vi "Dashboard Main.vi"() -> ()   [LabVIEW 2014]
uses:
  Program Files (x86)/National Instruments/LabVIEW 2014/examples/FRC/roboRIO/Vision/2015 Vision Example/Vision Support Code/Camera Types.ctl
  <vilib>/event_ctls.llb/eventvkey.ctl
  <vilib>/Rock Robotics/WPI/Dashboard/WPI_DashboardLogging Global.vi
  <vilib>/Rock Robotics/Network Tables/SD Write Number.vi
  <vilib>/Utility/config.llb/Write Key (String).vi
  <vilib>/Utility/config.llb/Write Key (I32).vi
  <vilib>/Utility/config.llb/NI_LVConfig.lvlib
  <vilib>/vision/NI_Vision_Development_Module.lvlib
panel:
  out "Camera Image 6":T1(plugin-control)
  in  "Tab Control":enum32{"Original", "Masked"}(tab)
  out "Original Image":T1(plugin-control)
  out "Masked":T1(plugin-control)
  out "Image Message":string="Timeout in Camera Communications"
  in  "TCP":refnum<k5>
  in  "Rec Mode":enum32{"Stop", "Record", "Playback"}(radio)
  in  "Vision":u16(ring)=3 items=["Camera Off", "USB Camera SW", "USB Camera HW", "IP Camera"]
  out "Camera IP":string
  in  "Dashboard Tab":T2(tab)
  in  "Camera Settings":T3={"Frame Rate"=30, "Compression"=30, "Size"=1} {"Frame Rate" scale=1.0..30.0; "Size" items=["640x480", "320x240", "160x120"]}
  out "MotorChart R":cluster{"Numeric":dbl, "Numeric":dbl}(graph)
  out "MotorChart L":T4(graph)
  out "MotorSliders R":cluster{"MotorSlide1":dbl, "MotorSlide2":dbl} {"MotorSlide2" scale=-1.0..1.0 scale format="%#_2e"; "MotorSlide1" scale=-1.0..1.0 scale format="%#_2e"}
  out "MotorSliders L":T5 {"MotorSlide4 2" scale=0.0..14.0 scale format="%#_2e"; "MotorSlide2" scale=-1.0..1.0 scale format="%#_2e"; "MotorSlide1" scale=-1.0..1.0 scale format="%#_2e"}
  out "Gyro":dbl(knob) scale=0.0..360.0
  out "JS1 Z":dbl(slide) scale=-1.0..1.0 scale format="%#_2e"
  out "JS1 Graph":cluster{"X":dbl, "Y":dbl}[](graph)
  out "JS1 Buttons":T6
  out "JS2 Z":dbl(slide) scale=-1.0..1.0 scale format="%#_2e"
  out "JS2 Graph":cluster{"X":dbl, "Y":dbl}[](graph)
  out "JS2 Buttons":T6
  out "Mode":T7(ring)=enum."Auto Disabled"
  in  "DB Camera Config":bool
  out "fps":dbl format="%#.1g"
  out "Mbps":dbl format="%#.1g"
  out "Mbps 2":bool
  out "Center":dbl
  out "Sorted Scores":T8(array[cluster]) {"Carpet" format="%#_3g"; "S" format="%#_3g"; "Trapezoid %" format="%#_3g"; "L" format="%#_3g"; "Area to CH" format="%#_3g"; "X" format="%#_3g"; "Y" format="%#_3g"}
  out "Detected Totes":T9(array[cluster]) {"Normalized Rect"."Numeric 5" format="%#_2g"; "Normalized Rect"."Numeric 3" format="%#_2g"; "Normalized Rect"."Numeric 2" format="%#_2g"; "Normalized Rect"."Numeric" format="%#_2g"}
  out "ms to process":u32
  in  "Tote Color":T10={"Hue"={23.67058792990901, 53.0}, "Sat"={88.0, 255.0}, "Val"={60.0, 159.85714285714286}} {"Hue" scale=0.0..255.0 scale format="%#_3g"}
  in  "Carpet Color":T11(tab)
  in  "Red":T10={"Hue"={231.0, 14.0}, "Sat"={83.0, 255.0}, "Val"={52.5, 255.0}} {"Hue" scale=0.0..255.0 scale format="%#_3g"}
  in  "Blue":T10={"Hue"={119.0, 181.0}, "Sat"={33.0, 255.0}, "Val"={48.571428571428584, 255.0}} {"Hue" scale=0.0..255.0 scale format="%#_3g"}
  in  "Annotate":bool=TRUE
  in  "Show Carpet Mask":bool=TRUE
  in  "Limit Tests?":bool=TRUE
  out "Particles":i32
  in  "Score Threshold":dbl=75.0
  in  "Aspect Fudge Factor":dbl=1.0
  in  "Camera Type":T12=enum."MS HD3000 square"
  out "Image":T1(plugin-control)
  in  "DB/String 9":string
  in  "DB/String 8":string
  in  "DB/String 7":string
  in  "DB/String 6":string
  in  "DB/String 5":string
  in  "DB/String 4":string
  in  "DB/String 3":string
  in  "DB/String 2":string
  in  "DB/String 1":string
  in  "DB/String 0":string
  in  "DB/Slider 0":dbl(slide) scale=0.0..5.0
  in  "DB/Slider 1":dbl(slide) scale=0.0..5.0
  in  "DB/Slider 2":dbl(slide) scale=0.0..5.0
  in  "DB/Slider 3":dbl(slide) scale=0.0..5.0
  out "DB/LED 3":bool
  out "DB/LED 2":bool
  out "DB/LED 1":bool
  out "DB/LED 0":bool
  in  "DB/Button 3":bool
  in  "DB/Button 2":bool
  in  "DB/Button 1":bool
  in  "DB/Button 0":bool caption="New Name"
  in  "Test Slider":dbl(slide) scale=0.0..100.0 scale format="%#_3g"
  in  "On/Off":bool caption="Solenoid"
  in  "Test Name":u16(ring) items=["Select the test to run...", "Example Test", "-------------------------------", "List of tests is built in robot code.", "Replace with your own automated tests."]
  in  "Test Tree":string(tree)
  in  "Motor":cluster{"Value":dbl, "Enable":bool} {"Value" scale=-1.0..1.0 scale format="%#_3g"}
  out "Progress":T13 {"Test Progress" scale=0.0..100.0}
  in  "Rev/Fwd":cluster{"Forward":bool, "Reverse":bool}
  in  "Test Ring":u16(ring) items=["Monochrome", "Color"]
  in  "Listbox":i32(listbox)
  out "Tree":string(tree)
  out "Boolean":bool
  # "Left"
  # "Front"
  # "Right"
  # "Battery"
  # "Density Profile"
  # "Aspect Ratio"
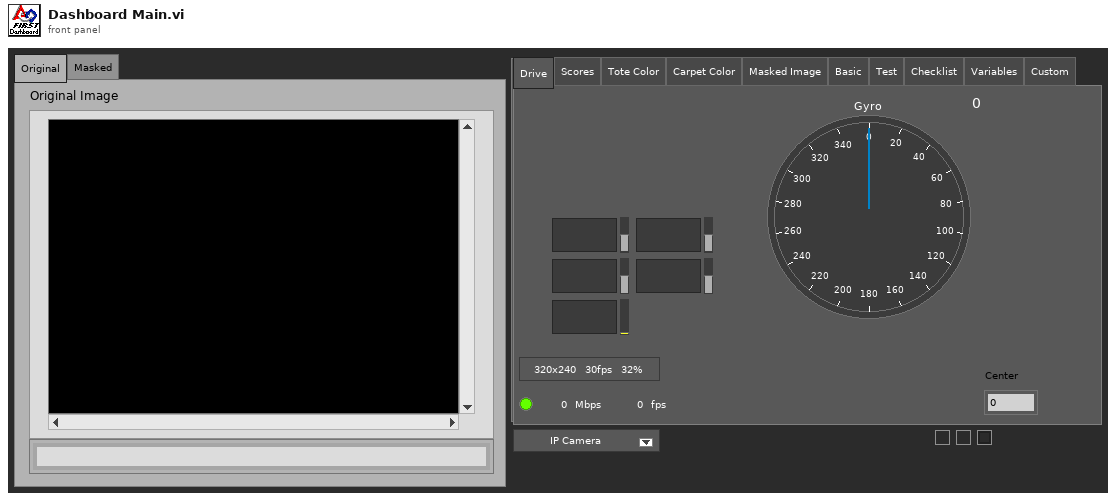
[diagram p1: front panel]
types:
  T1 = typedef "IMAQ Image.ctl" = refnum<image>
  T2 = enum32{"Drive", "Scores", "Tote Color", "Carpet Color", "Masked Image", "Basic", "Test", "Checklist", "Variables", "Custom"}
  T3 = cluster{"Frame Rate":i32, "Compression":i32, "Size":u16}
  T4 = cluster{"Numeric":dbl, "Numeric":dbl, "Battery V":dbl}
  T5 = cluster{"MotorSlide1":dbl, "MotorSlide2":dbl, "MotorSlide4 2":dbl}
  T6 = cluster{bool, bool, bool, bool, bool, bool, bool, bool, bool, bool, bool, bool}
  T7 = enum8{"Tele-Op Disabled", "Tele-Op Enabled", "Auto Disabled", "Auto Enabled", "Test Disabled", "Test Enabled", "Disconnected", "No Code", "E-Stop"}
  T8 = cluster{"Rectangle":cluster{"Numeric":dbl, "Numeric 2":dbl, "Numeric 3":dbl, "Numeric 5":dbl}, "Trapezoid %":dbl, "L":dbl, "S":dbl, "Area to CH":dbl, "X":dbl, "Y":dbl, "Carpet":dbl}[]
  T9 = cluster{"Distance (ft)":dbl, "Center":cluster{dbl, dbl}, "Normalized Rect":cluster{"Numeric":dbl, "Numeric 2":dbl, "Numeric 3":dbl, "Numeric 5":dbl}}[]
  T10 = cluster{"Hue":cluster{dbl, dbl}, "Sat":cluster{dbl, dbl}, "Val":cluster{dbl, dbl}}
  T11 = enum32{"Red Carpet Color", "Blue Carpet Color", "None"}
  T12 = typedef "Camera Types.ctl" = enum16{"206", "1011", "1013", "MS HD3000 square", "MS HD3000 640x480"}
  T13 = cluster{"Test Progress":u8, "Test Progress Text":string}
  T14 = typedef "Particle Parameters" = i32
  T15 = typedef "Image Type" = u32
  T16 = enum32{"Drive", "Basic", "Custom", "Test", "Checklist", "Variables"}
  T17 = cluster{"Camera Image 6":refnum<vi>, "Dashboard Tab":refnum<vi>, "Boolean":refnum<vi>, "Vision":refnum<vi>, "Rec Mode":refnum<vi>, "Test Slider":refnum<vi>, "On/Off ":refnum<vi>, "Test Ring":refnum<vi>, "Rev/Fwd":refnum<vi>, "Test Name":refnum<vi>, "Motor":refnum<vi>, "Progress":refnum<vi>, "CheckList":refnum<vi>, "Tree":refnum<vi>, "Test Tree":refnum<vi>}
  T18 = cluster{"Error Strings":string, "Disable Counts":cluster{u16, u16}, "Rail Faults":cluster{u16, u16, u16}, "Robot IP":string, "DB Mode":u8, "Event Info":cluster{"Name":string, "Type":u8, "Number":u16, "Replay":u8}, "Camera Addr":string}
  T19 = cluster{"Storage":cluster{"Disk Free":u64, "RAM Block":u32, "RAM free":u32}, "CPU Utilization":cluster{"CPU % ISR":sgl, "CPU % Time Crit":sgl, "CPU % Timed Str":sgl, "CPU % High":sgl, "CPU % Above":sgl, "CPU % Normal":sgl, "CPU % Low":sgl}, "CAN":cluster{"% Bus Utilization":sgl, "Bus Off Cnt":u32, "TX_FIFO Full Cnt":u32, "Receive Error Cnt":u8, "Transmit Error Cnt":u8}, "HID":cluster{"HID Outputs":u32, "Rumble Low":u16, "Rumble High":u16}[]}
  T20 = cluster{"Status bits":cluster{"Test Mode":bool, "Autonomous":bool, "Enabled":bool, "Code Start":bool, "Brownout":bool, "Reserved 2":bool, "Reserved 3":bool, "E-Stop":bool}, "Code Trace":cluster{"Disabled":bool, "TeleOp":bool, "Auto":bool, "Test":bool}, "Controller Type":enum16{"unknown", "cRIO", "roboRio"}, "Code?":enum16{"unknown", "noCode", "code"}, "Battery V":dbl}
  T21 = cluster{"Control Bits":cluster{"TestMode":bool, "Autonomous":bool, "Enabled":bool, "FMS Present":bool, bool, bool, bool, "E-Stop":bool}, "Team Station ":u8, "Countdown":sgl, "Joystick Values":cluster{"Axes":dbl[], "Buttons":bool[], "POVs":i16[]}[]}
  T22 = cluster{"Axes":dbl[], "Buttons":bool[], "POVs":i16[]}[]
  T23 = cluster{"Axes":dbl[], "Buttons":bool[], "POVs":i16[]}
  T24 = cluster{"Buttons[0]":bool, "Buttons[1]":bool, "Buttons[2]":bool, "Buttons[3]":bool, "Buttons[4]":bool, "Buttons[5]":bool, "Buttons[6]":bool, "Buttons[7]":bool, "Buttons[8]":bool, "Buttons[9]":bool, "Buttons[10]":bool, "Buttons[11]":bool}
  T25 = typedef "NI_LVConfig.lvlib/Config Data RefNum.ctl" = refnum<k1>
  T26 = cluster{"Operation":enum16{"Update", "Clear"}, "Color Box":u32}[]
  T27 = typedef "eventvkey.ctl" = enum16{"ASCII", "Enter", "Return", "Shift", "Ctrl", "Alt", "Cmd", "Opt", "Caps", "NumLock", "Clear", "Break", "Up", "Down", "Left", "Right", "Insert", "Delete", "Home", "End", "PageUp", "PageDown", "Escape", "Help", "Pause", "ScrollLock", "F1", "F2", "F3", "F4", "F5", "F6", "F7", "F8", "F9", "F10", "F11", "F12", "F13", "F14", "F15", "F16", "F17", "F18", "F19", "F20", "F21", "F22", "F23", "F24", "Play", "VolumeUp", "VolumeDown", "Mute", "Two Byte Char"}
  T28 = cluster{"Image Size":bool, "Image Type":bool, "Pixel Value":bool, "ROI Information":bool, "Zoom Factor":bool}
  T29 = enum8{"Enabled", "Disabled", "Disabled and Grayed Out"}
  T30 = cluster{"Operation":enum16{"Update", "Clear"}, "Color Box":u32}
  T31 = cluster{"Bounding box":cluster{"left":dbl, "top":dbl, "right":dbl, "bottom":dbl}, "Trapezoid":dbl, "Long Aspect":dbl, "Short Aspect":dbl, "Area to CH":dbl, "X Mask":dbl, "Y Mask":dbl, "Carpet":dbl}[]
  T32 = cluster{"Red":cluster{"Hue":cluster{dbl, dbl}, "Sat":cluster{dbl, dbl}, "Val":cluster{dbl, dbl}}, "Blue":cluster{"Hue":cluster{dbl, dbl}, "Sat":cluster{dbl, dbl}, "Val":cluster{dbl, dbl}}}
  T33 = cluster{cluster{"[0]":dbl, "[1]":dbl, "[2]":dbl, "[3]":dbl}, "Score":dbl, "Long Edge Score":dbl, "Short Edge Score":dbl, dbl, "X Score":dbl, "Y Score":dbl, "Carpet":dbl}[]
  T34 = cluster{"Found Totes[0]":cluster{"Distance (ft)":dbl, "Center":cluster{dbl, dbl}, "Normalized Rect":cluster{"Numeric":dbl, "Numeric 2":dbl, "Numeric 3":dbl, "Numeric 5":dbl}}, "Found Totes[1]":cluster{"Distance (ft)":dbl, "Center":cluster{dbl, dbl}, "Normalized Rect":cluster{"Numeric":dbl, "Numeric 2":dbl, "Numeric 3":dbl, "Numeric 5":dbl}}, "Found Totes[2]":cluster{"Distance (ft)":dbl, "Center":cluster{dbl, dbl}, "Normalized Rect":cluster{"Numeric":dbl, "Numeric 2":dbl, "Numeric 3":dbl, "Numeric 5":dbl}}, "Found Totes[3]":cluster{"Distance (ft)":dbl, "Center":cluster{dbl, dbl}, "Normalized Rect":cluster{"Numeric":dbl, "Numeric 2":dbl, "Numeric 3":dbl, "Numeric 5":dbl}}, "Found Totes[4]":cluster{"Distance (ft)":dbl, "Center":cluster{dbl, dbl}, "Normalized Rect":cluster{"Numeric":dbl, "Numeric 2":dbl, "Numeric 3":dbl, "Numeric 5":dbl}}, "Found Totes[5]":cluster{"Distance (ft)":dbl, "Center":cluster{dbl, dbl}, "Normalized Rect":cluster{"Numeric":dbl, "Numeric 2":dbl, "Numeric 3":dbl, "Numeric 5":dbl}}, "Found Totes[6]":cluster{"Distance (ft)":dbl, "Center":cluster{dbl, dbl}, "Normalized Rect":cluster{"Numeric":dbl, "Numeric 2":dbl, "Numeric 3":dbl, "Numeric 5":dbl}}, "Found Totes[7]":cluster{"Distance (ft)":dbl, "Center":cluster{dbl, dbl}, "Normalized Rect":cluster{"Numeric":dbl, "Numeric 2":dbl, "Numeric 3":dbl, "Numeric 5":dbl}}, "Found Totes[8]":cluster{"Distance (ft)":dbl, "Center":cluster{dbl, dbl}, "Normalized Rect":cluster{"Numeric":dbl, "Numeric 2":dbl, "Numeric 3":dbl, "Numeric 5":dbl}}}
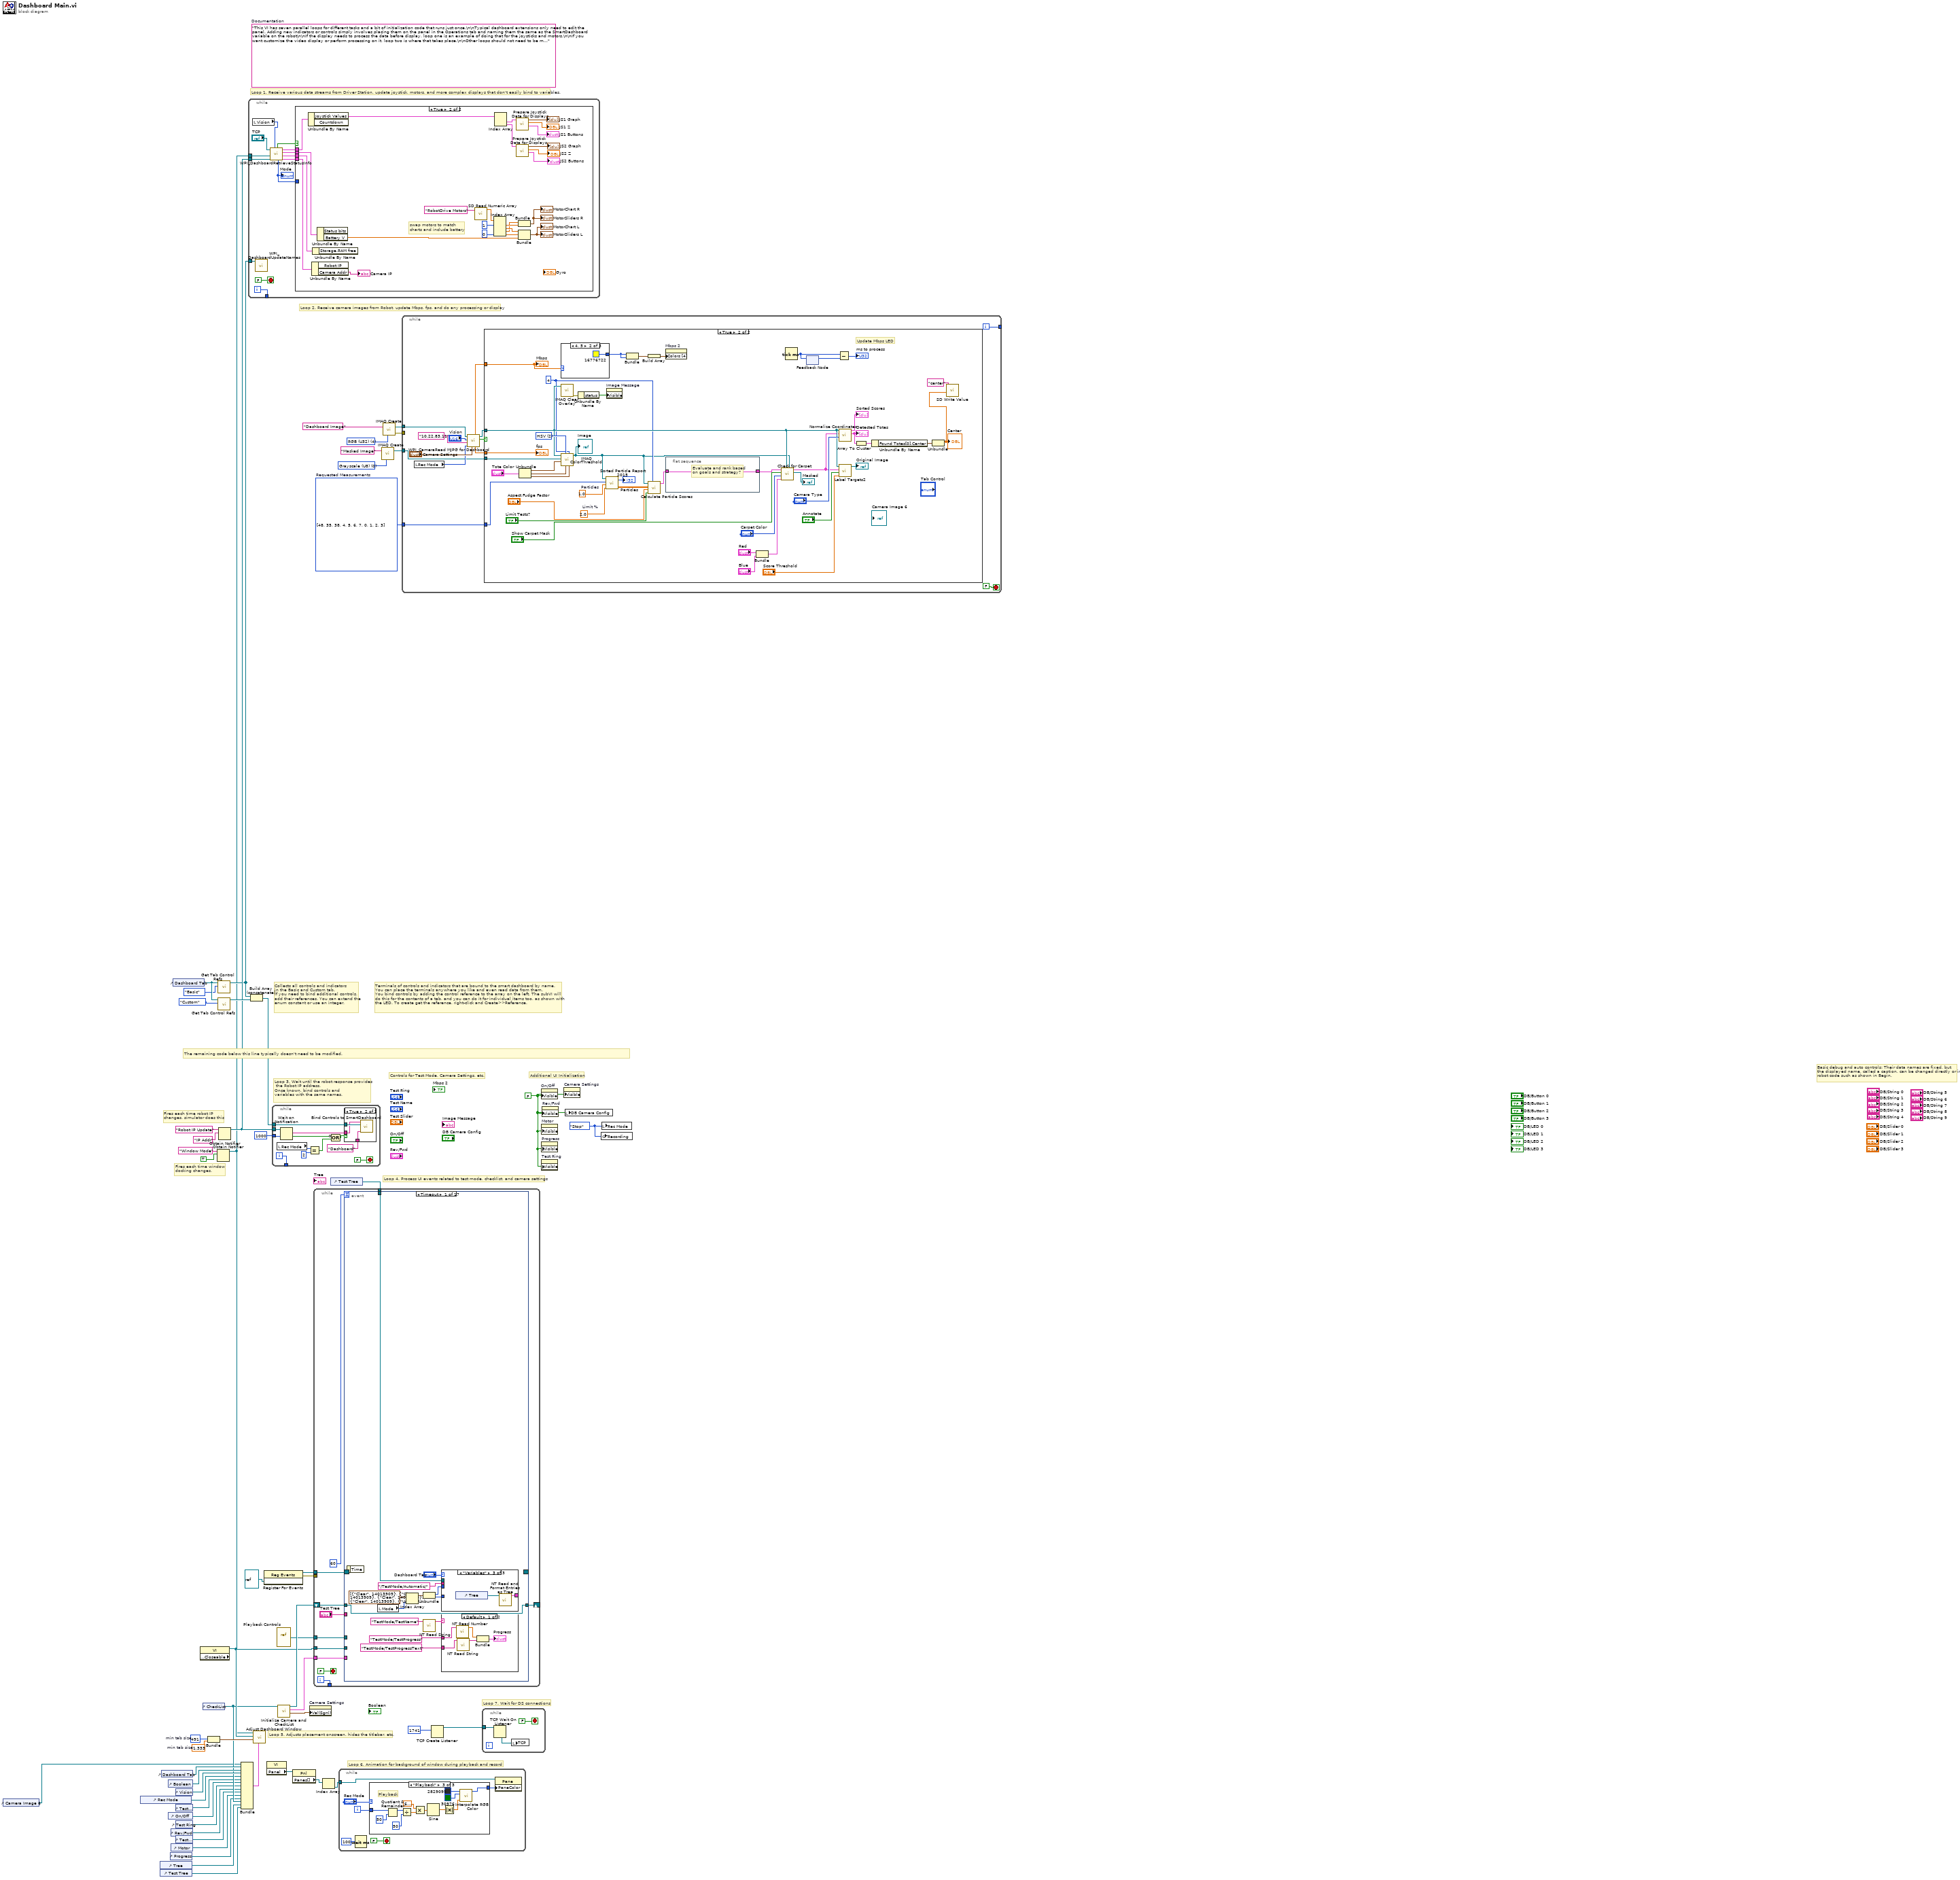
[diagram p0: block diagram]
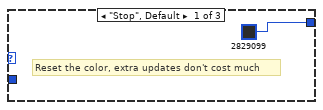
[diagram p3: hidden frame]
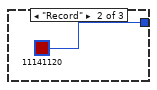
[diagram p4: hidden frame]
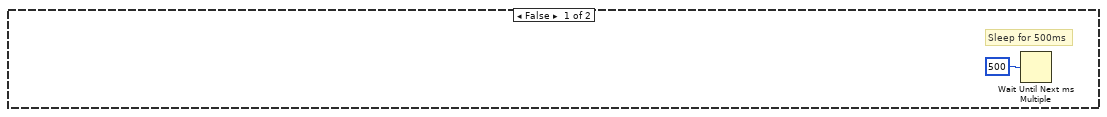
[diagram p6: hidden frame]
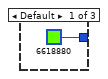
[diagram p7: hidden frame]
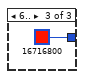
[diagram p8: hidden frame]
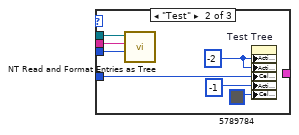
[diagram p10: hidden frame]
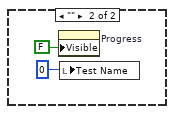
[diagram p11: hidden frame]
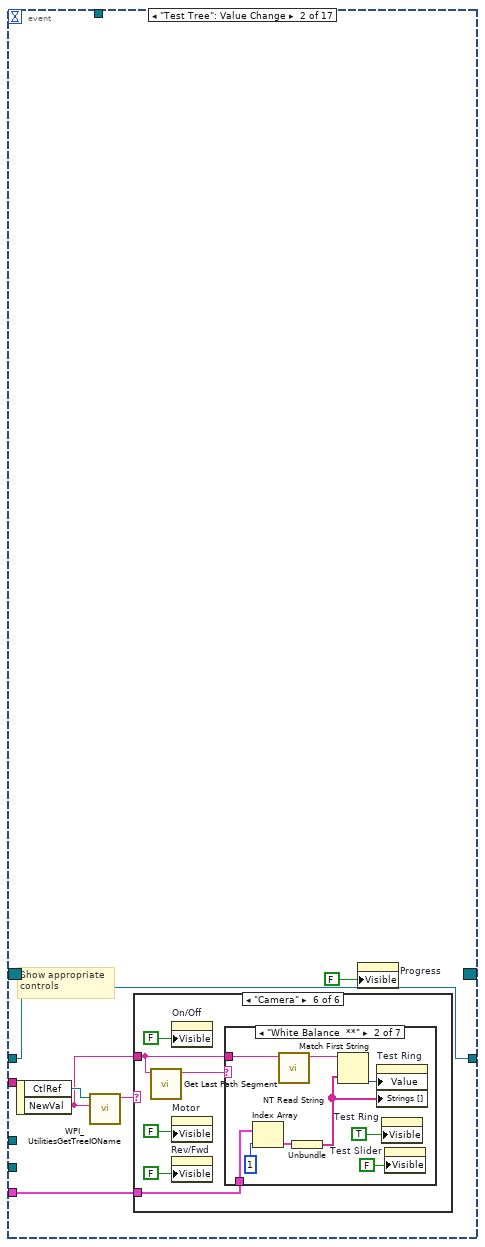
[diagram p12: hidden frame]
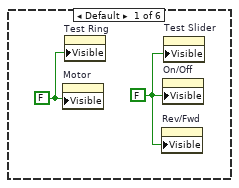
[diagram p13: hidden frame]
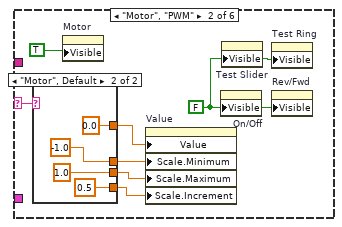
[diagram p14: hidden frame]
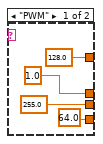
[diagram p15: hidden frame]
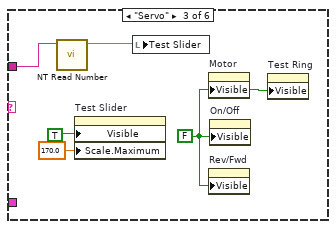
[diagram p16: hidden frame]
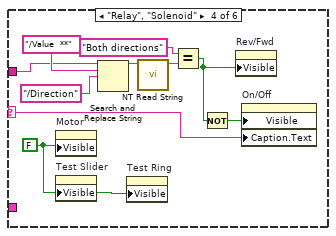
[diagram p17: hidden frame]
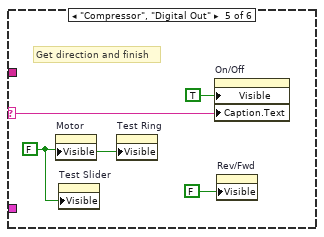
[diagram p18: hidden frame]
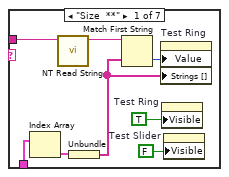
[diagram p19: hidden frame]
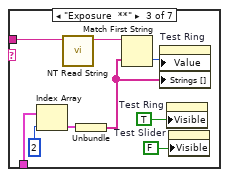
[diagram p20: hidden frame]
diagram:
  w3 = T14[] [48, 35, 38, 4, 5, 6, 7, 0, 1, 2, 3] items=["Center of Mass X", "Center of Mass Y", "First Pixel X", "First Pixel Y", "Bounding Rect Left", "Bounding Rect Top", "Bounding Rect Right", "Bounding Rect Bottom", "Max Feret Diameter Start X", "Max Feret Diameter Start Y", "Max Feret Diameter End X", "Max Feret Diameter End Y", "Max Horiz. Segment Length Left", "Max Horiz. Segment Length Right", "Max Horiz. Segment Length Row", "-", "Bounding Rect Width", "Bounding Rect Height", "Bounding Rect Diagonal", "Perimeter", "Convex Hull Perimeter", "Holes' Perimeter", "Max Feret Diameter", "Equivalent Ellipse Major Axis", "Equivalent Ellipse Minor Axis", "Equivalent Ellipse Minor Axis (Feret)", "Equivalent Rect Long Side", "Equivalent Rect Short Side", "Equivalent Rect Diagonal", "Equivalent Rect Short Side (Feret)", "Average Horiz. Segment Length", "Average Vert. Segment Length", "Hydraulic Radius", "Waddel Disk Diameter", "-", "Area", "Holes' Area", "Particle & Holes' Area", "Convex Hull Area", "Image Area", "-", "Number of Holes", "Number of Horiz. Segments", "Number of Vert. Segments", "-", "Orientation", "Max Feret Diameter Orientation", "-", "% Area/Image Area", "% Area/(Particle & Holes' Area)", "Ratio of Equivalent Ellipse Axes", "Ratio of Equivalent Rect Sides", "-", "Elongation Factor", "Compactness Factor", "Heywood Circularity Factor", "Type Factor", "-", "Sum X", "Sum Y", "Sum XX", "Sum XY", "Sum YY", "Sum XXX", "Sum XXY", "Sum XYY", "Sum YYY", "-", "Moment of Inertia XX", "Moment of Inertia XY", "Moment of Inertia YY", "Moment of Inertia XXX", "Moment of Inertia XXY", "Moment of Inertia XYY", "Moment of Inertia YYY", "Norm. Moment of Inertia XX", "Norm. Moment of Inertia XY", "Norm. Moment of Inertia YY", "Norm. Moment of Inertia XXX", "Norm. Moment of Inertia XXY", "Norm. Moment of Inertia XYY", "Norm. Moment of Inertia YYY", "Hu Moment 1", "Hu Moment 2", "Hu Moment 3", "Hu Moment 4", "Hu Moment 5", "Hu Moment 6", "Hu Moment 7"]  # Requested Measurements
  w6 = T15 0 items=["Grayscale (U8)", "Grayscale (I16)", "Grayscale (SGL)", "Complex (CSG)", "RGB (U32)", "HSL (U32)", "RGB (U64)"] ("Image Type")
  w30 = 491  # min tab size
  w29 = 1.333  # min tab size
  w37 = enum32{"Stop", "Record", "Playback"}."Stop" ("Rec Mode")
  w13 = FALSE ("Visible")
  (unwired) "This VI has seven parallel loops for different tasks and a bit of initialization code that runs just once.\n\nTypical dashboard extensions only need to edit the panel. Adding new indicators or controls simply involves placing them on the panel in the Operations tab and naming them the same as the SmartDashboard variable on the robot\n\nIf the display needs to process the data before display, loop one is an example of doing that for the joysticks and motors.\n\nIf you want customize the video display or perform processing on it, loop two is where that takes place.\n\nOther loops should not need to be modified. They are pretty standard, and document the task they perform."  # Documentation
  w56 = T15 4 items=["Grayscale (U8)", "Grayscale (I16)", "Grayscale (SGL)", "Complex (CSG)", "RGB (U32)", "HSL (U32)", "RGB (U64)"] ("Image Type")
  # "Loop 7. Wait for DS connections"
  # "Basic debug and auto controls: Their data names are fixed, but\nthe displayed name, called a caption, can be changed directly or in\nrobot code such as shown in Begin."
  # "Controls for Test Mode, Camera Settings, etc."
  # "Additional UI Initialization"
  # "Loop 6. Animation for background of window during playback and record"
  # "Fires each time robot IP\nchanges, simulator does this"
  # "Fires each time window\ndocking changes."
  # "Collects all controls and indicators\nin the Basic and Custom tab.\nIf you need to bind additional controls,\nadd their references. You can extend the\nenum constant or use an integer."
  # "The remaining code below this line typically doesn't need to be modified."
  # "Loop 4. Process UI events related to test mode, checklist, and camera settings"
  # "Terminals of controls and indicators that are bound to the smart dashboard by name.\nYou can place the terminals anywhere you like and even read data from them.\nYou bind controls by adding the control reference to the array on the left. The subVI will\ndo this for the contents of a tab, and you can do it for individual items too, as shown with\nthe LED. To create get the reference, right-click and Create>>Reference."
  # "Loop 3. Wait until the robot response provides\n the Robot IP address.\nOnce known, bind controls and\nvariables with the same names."
  # "Loop 5. Adjusts placement onscreen, hides the titlebar, etc."
  # "Loop 1. Receive various data streams from Driver Station, update joystick, motors, and more complex displays that don't easily bind to variables."
  # "Loop 2. Receive camera images from Robot, update Mbps, fps, and do any processing or display"
  n1 = control-ref of="Camera Image 6"() -> (w1:refnum<vi>)
  n2 = control-ref of="Rec Mode"() -> (w19:refnum<vi>)
  n3 = control-ref of="Tree"() -> (w23:refnum<vi>)
  n4 = control-ref of="Test Tree"() -> (w22:refnum<vi>)
  n5 = control-ref of="Dashboard Tab"() -> (w32:refnum<vi>)
  n6 = control-ref of="Boolean"() -> (w27:refnum<vi>)
  n7 = control-ref of="On/Off"() -> (w17:refnum<vi>)
  n8 = control-ref of="Progress"() -> (w14:refnum<vi>)
  n9 = control-ref of="Rev/Fwd"() -> (w15:refnum<vi>)
  n10 = control-ref of="Motor"() -> (w20:refnum<vi>)
  n11 = control-ref of="Dashboard Tab"() -> (w35:refnum<vi>)
  n12 = control-ref of="Test Slider"() -> (w18:refnum<vi>)
  n13 = control-ref of="Vision"() -> (w31:refnum<vi>)
  n14 = control-ref of="Test Ring"() -> (w16:refnum<vi>)
  n15 = control-ref of="Test Name"() -> (w21:refnum<vi>)
  n16 = property class="VI" props=["Front Panel.Closeable"]() -> (reference out=w36:refnum<vi>)  [unwired: 2 in, 2 out]
  n17 = control-ref of="CheckList"() -> (w24:refnum<vi>)
  n18 = Bundle("min tab size"=w30, "min tab size"=w29) -> (w28:cluster{"min tab size":i32, "min tab size":dbl})  [unwired: 1 in]
  n19 = Obtain Notifier(name (unnamed)="Window Mode", notification data type=TRUE) -> (notifier out=w10:refnum<notifier>)  [unwired: 2 in, 2 out]
  n20 = call <vilib>:"Get Tab Control Refs.vi"("Page Index"=T16."Basic" ("Dashboard Tab"), "TabControl in"=w35) -> ("ControlsOnPage"=w11:refnum<vi>[])  [unwired: 9 in]
  n21 = call <vilib>:"Get Tab Control Refs.vi"("Page Index"=T16."Custom" ("Dashboard Tab"), "TabControl in"=w35) -> ("ControlsOnPage"=w34:refnum<vi>[])  [unwired: 9 in]
  n22 = Obtain Notifier(name (unnamed)="Robot IP Update", notification data type="IP Addr" ("name (unnamed)")) -> (notifier out=w12:refnum<notifier>)  [unwired: 2 in, 2 out]
  n23 = Bundle("Camera Image 6"=w1, "Dashboard Tab"=w32, "Boolean"=w27, "Vision"=w31, "Rec Mode"=w19, "Test Slider"=w18, "On/Off"=w17, "Test Ring"=w16, "Rev/Fwd"=w15, "Test Name"=w21, "Motor"=w20, "Progress"=w14, "CheckList"=w24, "Tree"=w23, "Test Tree"=w22) -> (w2:T17)  [unwired: 1 in]
  n24 = while {
    tunnel: [w68] -> _
    tunnel: w12 -> [w62]
    tunnel: w11 -> [w61]
    tunnel: w10 -> [w57]
    i -> [w68]
    stop <- FALSE stop-if-true
    n25 = local read "Vision"() -> (w59:u16)
    n26 = call <vilib>:"WPI_DashboardUpdateNames.vi"("Controls on Tab"=w61) -> ()  [unwired: 11 in]
    n27 = call <vilib>:"WPI_DashboardRetrieveStatusInfo.vi"("Vision"=w59, "Binding Refnum"=w62, "Window Mode Notifier"=w57, "TCP Cnx"="TCP") -> ("Power and Errors"=w63:T18, "Robot Metrics"=w66:T19, "Status Info"=w67:T20, "Control Info"=w64:T21, "Robot Mode"=w60:T7, "Process?"=w65:bool)  [unwired: 2 in]
    "Mode" <- w60
    n28 = case shown="True" w65 {
      tunnel: w67 -> [_ w94]
      tunnel: w66 -> [_ w93]
      tunnel: w64 -> [_ w92]
      tunnel: w63 -> [_ w91]
      tunnel: w60 -> [_ _]
      frame False {
      }
      frame True {
        # "swap motors to match\ncharts and include battery"
        n29 = Unbundle By Name(w92) -> ("Joystick Values"=w79:T22)  [unwired: 1 out]
        n30 = Unbundle By Name(w91) -> ("Camera Addr"=→"Camera IP":string)  [unwired: 1 out]
        n31 = Unbundle By Name(w93) -> ()  [unwired: 1 out]
        n32 = Unbundle By Name(w94) -> ("Battery V"=w80:dbl)  [unwired: 1 out]
        n33 = call <vilib>:"SD Read Numeric Array.vi"("Name"="RobotDrive Motors") -> ("Numeric Array"=w82:dbl[])  [unwired: 8 in, 2 out]
        n34 = Index Array(array=w82, index #1=1, index #4=0) -> (element #1=w86:dbl, element #2=w87:dbl, element #3=w85:dbl, element #4=w90:dbl)  [unwired: 2 in]
        n35 = Index Array(array=w79) -> (element #1=w78:T23, element #2=w73:T23)  [unwired: 2 in]
        n36 = call "Prepare Joystick Data for Displays.vi"("Joystick Values"=w73) -> ("Buttons"=→"JS2 Buttons":T24, "Z Axis"=→"JS2 Z":dbl, "Cartesian Data"=→"JS2 Graph":cluster{"X axis":dbl, "X axis":dbl}[])  [unwired: 8 in]
        n37 = call "Prepare Joystick Data for Displays.vi"("Joystick Values"=w78) -> ("Buttons"=→"JS1 Buttons":T24, "Z Axis"=→"JS1 Z":dbl, "Cartesian Data"=→"JS1 Graph":cluster{"X axis":dbl, "X axis":dbl}[])  [unwired: 8 in]
        n38 = Bundle("Numeric"=w85, "Numeric"=w86) -> (→"MotorChart R" →"MotorSliders R":cluster{"Numeric":dbl, "Numeric":dbl})  [unwired: 1 in]
        n39 = Bundle("Numeric"=w87, "Numeric"=w90, "Battery V"=w80) -> (→"MotorChart L" →"MotorSliders L":T4)  [unwired: 1 in]
      }
    }
  }
  n40 = Build Array (concatenate)(w11, w34) -> (w33:refnum<vi>[])
  n41 = call "Adjust Dashboard Window.vi"("Sizing Refnums"=w2, "Size Constraints"=w28, "VI"=w36, "Notifier in"=w10) -> ()  [unwired: 8 in]
  n42 = register-events(refnum<vi> refnum) -> (reference out=w41:refnum<event-registration>, error out=w40:errorcluster)  [unwired: 2 in]
  n43 = property class="VI"() -> ("Panel"=w44:refnum<vi>)  [unwired: 2 in, 2 out]
  n44 = while {
    tunnel: w33 -> [w106]
    tunnel: w12 -> [w104]
    tunnel: [w102] -> _
    tunnel: u32 1000 ("milliseconds to wait") -> [w101]
    i -> [w102]
    stop <- FALSE stop-if-true
    n45 = local read "Rec Mode"() -> (w97:enum32{"Stop", "Record", "Playback"})
    n46 = Wait on Notification(notifier=w104, timeout in ms (-1)=w101) -> (notification=w103:string, timed out?=w99:bool)  [unwired: 2 in, 2 out]
    n47 = Equal?(x=w97, y=u16 2 ("Rec Mode")) -> (x = y?=w98:bool)
    n48 = Compound Arithmetic op=OR(invert w99, w98) -> (w100:bool)
    n49 = case shown="True" w100 {
      tunnel: w106 -> [_ w109]
      tunnel: w103 -> [_ w108]
      tunnel: "Dashboard" -> [_ w107]
      frame False {
      }
      frame True {
        n50 = call <vilib>:"Bind Controls to SmartDashboard.vi"("Client Name"=w107, "Bound Control Refs"=w109, "Server IP Address"=w108) -> ()  [unwired: 9 in]
      }
    }
  }
  n51 = vi-ref "Playback Controls.vi"() -> (w42:refnum<vi>)
  n52 = call "Initialize Camera and CheckList.vi"("ListBox in"=w24) -> ("Cluster"=w48:cluster{"value":i32, "value":i32, "index":i32}, "Array"=w49:cluster{string[]}[], "File Refnum"=w47:T25)  [unwired: 8 in]
  n53 = property class="Pnl"(reference=w44) -> ("Panes[]"=w45:refnum<vi>[])  [unwired: 1 in, 2 out]
  n54 = property on="Camera Settings" class="Clust (strict)"("Val(Sgnl)"=w48) -> ()  [unwired: 2 in, 2 out]
  n55 = Index Array(array=w45) -> (element=w43:refnum<vi>)  [unwired: 1 in]
  n56 = control-ref of="Test Tree"() -> (w46:refnum<vi>)
  n57 = while {
    tunnel: w49 -> [w117]
    shift-right: [w116] -> _
    shift-left: w47 -> [w115]
    tunnel: [w114] -> _
    tunnel: w46 -> [w113]
    tunnel: w42 -> [w112]
    tunnel: w41 -> [w111]
    tunnel: w40 -> [_]
    tunnel: w36 -> [w110]
    i -> [w114]
    stop <- FALSE stop-if-true
    n58 = event shown="[0] Timeout" {
      selector: w111 -> [_ _ _ _ _ _ _ _ _ _ _ _ _ _ _ _ _]
      dyn-events: [_ _ _ _ _ _ _ _ _ _ _ _ _ w353 _ _ _] -> _
      timeout: u32 60 ("milliseconds to wait") -> [_ _ _ _ _ _ _ _ _ _ _ _ _ _ _ _ _]
      tunnel: w113 -> [w129 _ _ _ _ _ _ _ _ _ _ _ _ _ _ _ _]
      tunnel: "Test Tree" -> [_ _ _ _ _ _ _ _ w324 w332 w334 w338 w346 _ _ _ _]
      tunnel: w117 -> [_ w151 _ _ _ _ w288 w318 _ _ _ _ _ _ _ _ _]
      tunnel: [w125 w150 w249 w254 w262 w274 w287 w311 w323 w330 w333 w337 w345 w355 w369 w370 w380] -> w116
      tunnel: w115 -> [w125 w150 w249 w254 w262 w274 w286 w311 w323 w330 w333 w337 w345 w355 w369 w370 w380]
      tunnel: w112 -> [_ _ _ _ _ _ _ _ _ _ _ _ _ w356 _ w373 _]
      tunnel: w110 -> [_ _ _ _ _ _ _ _ _ _ _ _ _ w351 _ _ _]
      event Timeout {
        n59 = event-data() -> ()  [unwired: 1 in, 1 out]
        n60 = local read "Mode"() -> (w128:T7)
        n61 = Index Array(array=T26 [{"Operation"=enum."Clear", "Color Box"=14013909}, {"Operation"=enum."Clear", "Color Box"=14013909}, {"Operation"=enum."Clear", "Color Box"=14013909}, {"Operation"=enum."Clear", "Color Box"=14013909}, {"Operation"=enum."Update", "Color Box"=14013909}, {"Operation"=enum."Update", "Color Box"=16777215}, {"Operation"=enum."Clear", "Color Box"=14013909}, {"Operation"=enum."Clear", "Color Box"=14013909}, {"Operation"=enum."Clear", "Color Box"=14013909}], index=w128) -> (element=w123:T30)
        n62 = Unbundle(w123) -> ("Operation"=w122:enum16{"Update", "Clear"}, "Color Box"=w121:u32)
        n63 = call <vilib>:"NT Read String.vi"("Name"="TestMode/TestName") -> ("String"=w132:string)  [unwired: 9 in, 1 out]
        n64 = case shown="\"Variables\"" "Dashboard Tab" {
          tunnel: w129 -> [_ w140 _]
          tunnel: "/TestMode/Automatic/" ("Name Pattern") -> [_ w139 _]
          tunnel: w122 -> [_ w138 _]
          tunnel: [_ _ w142] -> _
          tunnel: w121 -> [_ w134 _]
          frame "Custom", Default {
          }
          frame "Test" {
            w137 = -2 ("Active Item:Row Number")
            n65 = call <vilib>:"NT Read and Format Entries as Tree.vi"("Operation"=w138, "Name Pattern"=w139, "Tree Refnum"=w140) -> ()  [unwired: 7 in, 2 out]
            n66 = property on="Test Tree" class="Tree (strict)"("Active Item Row Number"=w137, "ActiveColNum"=w137, "CellBG"=w134, "Active Item Row Number"=-1 ("Active Item:Row Number"), "CellBG"=u32 5789784 ("Color Box")) -> ()  [unwired: 2 in, 2 out]
          }
          frame "Variables" {
            n67 = control-ref of="Tree"() -> (w141:refnum<vi>)
            n68 = call <vilib>:"NT Read and Format Entries as Tree.vi"("Tree Refnum"=w141) -> ("Formatted Strings"=w142:cluster{"Name":string, "Value":string}[])  [unwired: 9 in, 1 out]
          }
        }
        n69 = case shown="Default" w132 {
          tunnel: "TestMode/TestProgress" ("Name") -> [w144 _]
          tunnel: "TestMode/TestProgressText" ("Name") -> [w143 _]
          frame Default {
            n70 = call <vilib>:"NT Read Number.vi"("Name"=w144) -> ("Numeric"=w145:dbl)  [unwired: 9 in, 1 out]
            n71 = call <vilib>:"NT Read String.vi"("Name"=w143) -> ("String"=w146:string)  [unwired: 9 in, 1 out]
            n72 = Bundle("Numeric"=w145, "String"=w146) -> (→"Progress":cluster{"Numeric":dbl, "String":string})  [unwired: 1 in]
          }
          frame "" {
            n73 = property on="Progress" class="Clust (strict)"("Visible"=FALSE) -> ()  [unwired: 2 in, 2 out]
            n74 = local write "Test Name"(u16 0) -> ()
          }
        }
      }
      event "Test Tree": Value Change {
        # "Show appropriate\ncontrols"
        n75 = event-data() -> ("CtlRef"=w154:refnum<vi>, "NewVal"=w152:string)  [unwired: 1 in]
        n76 = call <vilib>:"WPI_UtilitiesGetTreeIOName.vi"("NewVal"=w152, "TreeControl in"=w154) -> ("I/O Name"=w155:string)  [unwired: 9 in]
        n77 = case shown="\"Camera\"" w155 {
          selector: w155 -> [_ w162 _ w180 w189 _]
          tunnel: w152 -> [_ _ w177 w179 _ w196]
          tunnel: w151 -> [_ _ _ _ _ w195]
          frame Default {
            w157 = FALSE ("Visible")
            w156 = FALSE ("Visible")
            n78 = property on="Motor" class="Clust (strict)"("Visible"=w156) -> ()  [unwired: 2 in, 2 out]
            n79 = property on="Test Ring" class="Ring (strict)"("Visible"=w156) -> ()  [unwired: 2 in, 2 out]
            n80 = property on="Rev/Fwd" class="Clust (strict)"("Visible"=w157) -> ()  [unwired: 2 in, 2 out]
            n81 = property on="On/Off" class="Bool (strict)"("Visible"=w157) -> ()  [unwired: 2 in, 2 out]
            n82 = property on="Test Slider" class="Slide (strict)"("Visible"=w157) -> ()  [unwired: 2 in, 2 out]
          }
          frame "Motor", "PWM" {
            w163 = FALSE ("Visible")
            n83 = case shown="\"Motor\", Default" w162 {
              tunnel: [1.0 ("Value") -1.0 ("Value")] -> w161
              tunnel: [255.0 ("Value") 1.0 ("Value")] -> w160
              tunnel: [128.0 ("Value") 0.0 ("Value")] -> w159
              tunnel: [64.0 ("Value") 0.5 ("Value")] -> w158
              frame "PWM" {
              }
              frame "Motor", Default {
              }
            }
            n84 = property on="Motor" class="Clust (strict)"("Visible"=TRUE) -> ()  [unwired: 2 in, 2 out]
            n85 = property on="Value" class="Slide (strict)"("Value"=w159, "Scale.Minimum"=w161, "Scale.Maximum"=w160, "Scale.Increment"=w158) -> ()  [unwired: 2 in, 2 out]
            n86 = property on="On/Off" class="Bool (strict)"("Visible"=w163) -> ()  [unwired: 2 in, 2 out]
            n87 = property on="Test Slider" class="Slide (strict)"("Visible"=w163) -> ()  [unwired: 2 in, 2 out]
            n88 = property on="Test Ring" class="Ring (strict)"("Visible"=w163) -> ()  [unwired: 2 in, 2 out]
            n89 = property on="Rev/Fwd" class="Clust (strict)"("Visible"=w163) -> ()  [unwired: 2 in, 2 out]
          }
          frame "Servo" {
            w175 = FALSE ("Visible")
            n90 = call <vilib>:"NT Read Number.vi"("Name"=w177) -> ("Numeric"=w176:dbl)  [unwired: 9 in, 1 out]
            n91 = property on="Test Slider" class="Slide (strict)"("Visible"=TRUE, "Scale.Maximum"=170.0 ("Scale.Range:Maximum")) -> ()  [unwired: 2 in, 2 out]
            n92 = local write "Test Slider"(w176) -> ()
            n93 = property on="Motor" class="Clust (strict)"("Visible"=w175) -> ()  [unwired: 2 in, 2 out]
            n94 = property on="Rev/Fwd" class="Clust (strict)"("Visible"=w175) -> ()  [unwired: 2 in, 2 out]
            n95 = property on="On/Off" class="Bool (strict)"("Visible"=w175) -> ()  [unwired: 2 in, 2 out]
            n96 = property on="Test Ring" class="Ring (strict)"("Visible"=w175) -> ()  [unwired: 2 in, 2 out]
          }
          frame "Relay", "Solenoid" {
            w178 = FALSE ("Visible")
            n97 = property on="Motor" class="Clust (strict)"("Visible"=w178) -> ()  [unwired: 2 in, 2 out]
            n98 = property on="Test Slider" class="Slide (strict)"("Visible"=w178) -> ()  [unwired: 2 in, 2 out]
            n99 = Search and Replace String(input string=w179, search string="/Value  **", replace string="/Direction") -> (result string=w185:string)  [unwired: 5 in, 3 out]
            n100 = property on="Test Ring" class="Ring (strict)"("Visible"=w178) -> ()  [unwired: 2 in, 2 out]
            n101 = call <vilib>:"NT Read String.vi"("Name"=w185) -> ("String"=w183:string)  [unwired: 9 in, 1 out]
            n102 = Equal?(x="Both directions", y=w183) -> (x = y?=w181:bool)
            n103 = Not(x=w181) -> (.not. x?=w182:bool)
            n104 = property on="Rev/Fwd" class="Clust (strict)"("Visible"=w181) -> ()  [unwired: 2 in, 2 out]
            n105 = property on="On/Off" class="Bool (strict)"("Visible"=w182, "Caption.Text"=w180) -> ()  [unwired: 2 in, 2 out]
          }
          frame "Compressor", "Digital Out" {
            w188 = FALSE ("Visible")
            # "Get direction and finish"
            n106 = property on="Motor" class="Clust (strict)"("Visible"=w188) -> ()  [unwired: 2 in, 2 out]
            n107 = property on="Test Slider" class="Slide (strict)"("Visible"=w188) -> ()  [unwired: 2 in, 2 out]
            n108 = property on="Test Ring" class="Ring (strict)"("Visible"=w188) -> ()  [unwired: 2 in, 2 out]
            n109 = property on="On/Off" class="Bool (strict)"("Visible"=TRUE, "Caption.Text"=w189) -> ()  [unwired: 2 in, 2 out]
            n110 = property on="Rev/Fwd" class="Clust (strict)"("Visible"=FALSE) -> ()  [unwired: 2 in, 2 out]
          }
          frame "Camera" {
            n111 = call <vilib>:"Get Last Path Segment.vi"("String in"=w196) -> ("String out"=w197:string)  [unwired: 10 in]
            n112 = property on="On/Off" class="Bool (strict)"("Visible"=FALSE) -> ()  [unwired: 2 in, 2 out]
            n113 = property on="Motor" class="Clust (strict)"("Visible"=FALSE) -> ()  [unwired: 2 in, 2 out]
            n114 = property on="Rev/Fwd" class="Clust (strict)"("Visible"=FALSE) -> ()  [unwired: 2 in, 2 out]
            n115 = case shown="\"White Balance  **\"" w197 {
              tunnel: w196 -> [w203 w212 w221 w230 w239 _ w245]
              tunnel: w195 -> [w201 w209 w218 w227 w236 _ _]
              frame "Size  **" {
                n116 = Index Array(array=w201) -> (element=w200:cluster{string[]})  [unwired: 1 in]
                n117 = call <vilib>:"NT Read String.vi"("Name"=w203) -> ("String"=w202:string)  [unwired: 9 in, 1 out]
                n118 = Unbundle(w200) -> (w198:string[])
                n119 = Match First String(2:w198, 3:w202) -> (0:w199:i32)  [unwired: 1 out]
                n120 = property on="Test Ring" class="Ring (strict)"("Value"=w199, "Strings []"=w198) -> ()  [unwired: 2 in, 2 out]
                n121 = property on="Test Ring" class="Ring (strict)"("Visible"=TRUE) -> ()  [unwired: 2 in, 2 out]
                n122 = property on="Test Slider" class="Slide (strict)"("Visible"=FALSE) -> ()  [unwired: 2 in, 2 out]
              }
              frame "White Balance  **" {
                n123 = Index Array(array=w209, index=1) -> (element=w210:cluster{string[]})
                n124 = call <vilib>:"NT Read String.vi"("Name"=w212) -> ("String"=w211:string)  [unwired: 9 in, 1 out]
                n125 = Unbundle(w210) -> (w207:string[])
                n126 = Match First String(2:w207, 3:w211) -> (0:w206:i32)  [unwired: 1 out]
                n127 = property on="Test Ring" class="Ring (strict)"("Value"=w206, "Strings []"=w207) -> ()  [unwired: 2 in, 2 out]
                n128 = property on="Test Ring" class="Ring (strict)"("Visible"=TRUE) -> ()  [unwired: 2 in, 2 out]
                n129 = property on="Test Slider" class="Slide (strict)"("Visible"=FALSE) -> ()  [unwired: 2 in, 2 out]
              }
              frame "Exposure  **" {
                n130 = Index Array(array=w218, index=2) -> (element=w219:cluster{string[]})
                n131 = call <vilib>:"NT Read String.vi"("Name"=w221) -> ("String"=w220:string)  [unwired: 9 in, 1 out]
                n132 = Unbundle(w219) -> (w215:string[])
                n133 = Match First String(2:w215, 3:w220) -> (0:w216:i32)  [unwired: 1 out]
                n134 = property on="Test Ring" class="Ring (strict)"("Value"=w216, "Strings []"=w215) -> ()  [unwired: 2 in, 2 out]
                n135 = property on="Test Ring" class="Ring (strict)"("Visible"=TRUE) -> ()  [unwired: 2 in, 2 out]
                n136 = property on="Test Slider" class="Slide (strict)"("Visible"=FALSE) -> ()  [unwired: 2 in, 2 out]
              }
              frame "Exposure Priority  **" {
                n137 = Index Array(array=w227, index=3) -> (element=w228:cluster{string[]})
                n138 = call <vilib>:"NT Read String.vi"("Name"=w230) -> ("String"=w229:string)  [unwired: 9 in, 1 out]
                n139 = Unbundle(w228) -> (w224:string[])
                n140 = Match First String(2:w224, 3:w229) -> (0:w225:i32)  [unwired: 1 out]
                n141 = property on="Test Ring" class="Ring (strict)"("Value"=w225, "Strings []"=w224) -> ()  [unwired: 2 in, 2 out]
                n142 = property on="Test Ring" class="Ring (strict)"("Visible"=TRUE) -> ()  [unwired: 2 in, 2 out]
                n143 = property on="Test Slider" class="Slide (strict)"("Visible"=FALSE) -> ()  [unwired: 2 in, 2 out]
              }
              frame "Color Enable  **" {
                n144 = Index Array(array=w236, index=4) -> (element=w237:cluster{string[]})
                n145 = call <vilib>:"NT Read String.vi"("Name"=w239) -> ("String"=w238:string)  [unwired: 9 in, 1 out]
                n146 = Unbundle(w237) -> (w233:string[])
                n147 = Match First String(2:w233, 3:w238) -> (0:w234:i32)  [unwired: 1 out]
                n148 = property on="Test Ring" class="Ring (strict)"("Value"=w234, "Strings []"=w233) -> ()  [unwired: 2 in, 2 out]
                n149 = property on="Test Ring" class="Ring (strict)"("Visible"=TRUE) -> ()  [unwired: 2 in, 2 out]
                n150 = property on="Test Slider" class="Slide (strict)"("Visible"=FALSE) -> ()  [unwired: 2 in, 2 out]
              }
              frame Default {
                n151 = property on="Test Ring" class="Ring (strict)"("Visible"=FALSE) -> ()  [unwired: 2 in, 2 out]
                n152 = property on="Test Slider" class="Slide (strict)"("Visible"=FALSE) -> ()  [unwired: 2 in, 2 out]
              }
              frame "Brightness  **", "Color Level  **", "Compression  **", "FPS  **", "Sharpness  **" {
                n153 = call <vilib>:"NT Read Number.vi"("Name"=w245) -> ("Numeric"=w244:dbl)  [unwired: 9 in, 1 out]
                n154 = local write "Test Slider"(w244) -> ()
                n155 = property on="Test Slider" class="Slide (strict)"("Visible"=TRUE, "Scale.Maximum"=100.0 ("Scale.Range:Maximum")) -> ()  [unwired: 2 in, 2 out]
                n156 = property on="Test Ring" class="Ring (strict)"("Visible"=FALSE) -> ()  [unwired: 2 in, 2 out]
              }
            }
          }
        }
        n157 = property on="Progress" class="Clust (strict)"("Visible"=FALSE) -> ()  [unwired: 2 in, 2 out]
      }
      event "Test Name": Mouse Enter {
        # "Populate the ring with the list of tests"
        n158 = event-data() -> ()  [unwired: 1 in, 1 out]
        n159 = call <vilib>:"NT Read String Array.vi"("Name"="TestMode/TestList") -> ("String Array"=w253:string[])  [unwired: 9 in, 1 out]
        n160 = Build Array (concatenate)("Select the test to run...", w253) -> (w252:string[])
        n161 = property on="Test Name" class="Ring (strict)"("Strings []"=w252) -> ()  [unwired: 2 in, 2 out]
      }
      event "Test Name": Value Change {
        w255 = FALSE ("Visible")
        # "Tell the robot the test name to run"
        n162 = event-data() -> ("NewVal"=w259:u16)  [unwired: 1 in]
        n163 = property on="Test Name" class="Ring (strict)"() -> ("Strings []"=w260:string[])  [unwired: 2 in, 2 out]
        n164 = local write "Progress"(T13 {"Test Progress"=0, "Test Progress Text"=""} ("Progress")) -> ()
        n165 = Index Array(array=w260, index=w259) -> (element=w258:string)
        n166 = call <vilib>:"NT Write String.vi"("String"=w258, "Name"="TestMode/TestName") -> ()  [unwired: 9 in, 1 out]
        n167 = property on="Progress" class="Clust (strict)"("Visible"=TRUE) -> ()  [unwired: 2 in, 2 out]
        n168 = property on="Motor" class="Clust (strict)"("Visible"=w255) -> ()  [unwired: 2 in, 2 out]
        n169 = property on="Test Slider" class="Slide (strict)"("Visible"=w255) -> ()  [unwired: 2 in, 2 out]
        n170 = property on="On/Off" class="Bool (strict)"("Visible"=w255) -> ()  [unwired: 2 in, 2 out]
        n171 = property on="Rev/Fwd" class="Clust (strict)"("Visible"=w255) -> ()  [unwired: 2 in, 2 out]
        n172 = property on="Test Ring" class="Ring (strict)"("Visible"=w255) -> ()  [unwired: 2 in, 2 out]
      }
      event "Listbox": Double Click {
        # "Shift clears all"
        # "Update symbols on the listbox"
        n173 = event-data() -> ("PlatMods.Shift"=w263:bool, "Row"=w265:i32)  [unwired: 1 in]
        n174 = case shown="True" w263 {
          tunnel: w265 -> [w269 _]
          tunnel: 1 -> [w268 _]
          frame False {
            n175 = property on="Listbox" class="LstBox (strict)"() -> ("Item Symbols"=w267:i32[])  [unwired: 2 in, 2 out]
            n176 = Replace Array Subset(array=w267, new element=w268, index=w269) -> (w266:i32[])
            n177 = property on="Listbox" class="LstBox (strict)"("Item Symbols"=w266) -> ()  [unwired: 2 in, 2 out]
          }
          frame True {
            w270 = 0 ("Top Row")
            n178 = property on="Listbox" class="LstBox (strict)"() -> ("Number of Rows"=w272:u32)  [unwired: 2 in, 2 out]
            n179 = Initialize Array(0, w272) -> (w271:i32[])
            n180 = property on="Listbox" class="LstBox (strict)"("Top Row"=w270, "Value"=w270, "Item Symbols"=w271) -> ()  [unwired: 2 in, 2 out]
          }
        }
      }
      event "Listbox": Key Down {
        # "Update symbols on the listbox\nLeft and right keys check and uncheck"
        n181 = event-data() -> ("VKey"=w276:T27)  [unwired: 1 in]
        n182 = case shown="\"Left\", \"Right\"" w276 {
          selector: w276 -> [w281 _]
          tunnel: eventvkey."Left" ("VKey") -> [w279 _]
          frame "Left", "Right" {
            n183 = Equal?(x=w279, y=w281) -> (x = y?=w280:bool)
            n184 = Select(t=0, s=w280, f=1) -> (s? t:f=w282:i32)
            n185 = property on="Listbox" class="LstBox (strict)"() -> ("Item Symbols"=w285:i32[])  [unwired: 2 in, 2 out]
            n186 = Replace Array Subset(array=w285, new element=w282, index="Listbox") -> (w284:i32[])
            n187 = property on="Listbox" class="LstBox (strict)"("Item Symbols"=w284) -> ()  [unwired: 2 in, 2 out]
          }
          frame Default {
          }
        }
      }
      event "DB Camera Config": Value Change {
        # "Show or hide the cluster of controls, store in ini file"
        n188 = event-data() -> ("NewVal"=w289:bool)  [unwired: 1 in]
        n189 = case shown="False" w289 {
          tunnel: w288 -> [w298 _]
          tunnel: [w291 w309] -> w287
          tunnel: w286 -> [w290 w309]
          frame False {
            w305 = "Camera"
            w308 = FALSE ("Visible")
            n190 = local read "Camera Settings"() -> (w297:T3)
            n191 = Index Array(array=w298) -> (element=w301:cluster{string[]})  [unwired: 1 in]
            n192 = Unbundle(w297) -> ("Frame Rate"=w296:i32, "Compression"=w295:i32, "Size"=w299:u16)
            n193 = Unbundle(w301) -> (w300:string[])
            n194 = Index Array(array=w300, index=w299) -> (element=w294:string)
            n195 = call-poly <vilib>:"Write Key.vi"("section"=w305, "value"=w294, "key"="Size", "refnum"=w290) -> ("refnum out"=w307:T25)  [unwired: 2 in, 5 out]
            n196 = call-poly <vilib>:"Write Key.vi"("section"=w305, "value"=w296, "key"="FrameRate", "refnum"=w307) -> ("refnum out"=w306:T25)  [unwired: 1 in, 6 out]
            n197 = property on="Camera Settings" class="Clust (strict)"("Visible"=w308) -> ()  [unwired: 2 in, 2 out]
            n198 = local write "DB Camera Config"(w308) -> ()
            n199 = call-poly <vilib>:"Write Key.vi"("section"=w305, "value"=w295, "key"="Compression", "refnum"=w306) -> ("refnum out"=w292:T25)  [unwired: 1 in, 6 out]
            n200 = call <vilib>:"Close Config Data.vi"("refnum"=w292) -> ("file path"=w293:path)  [unwired: 2 in, 8 out]
            n201 = call <vilib>:"Open Config Data.vi"("configuration file path"=w293) -> ("refnum"=w291:T25)  [unwired: 8 in, 2 out]
          }
          frame True {
            n202 = property on="Camera Settings" class="Clust (strict)"("Visible"=TRUE) -> ()  [unwired: 2 in, 2 out]
          }
        }
      }
      event "Camera Settings": Value Change {
        # "Update summary string when any elements of DB camera change"
        n203 = event-data() -> ("NewVal"=w322:T3)  [unwired: 1 in]
        n204 = Index Array(array=w318) -> (element=w317:cluster{string[]})  [unwired: 1 in]
        n205 = Unbundle(w322) -> ("Frame Rate"=w313:i32, "Compression"=w312:i32, "Size"=w315:u16)
        n206 = Unbundle(w317) -> (w316:string[])
        n207 = Index Array(array=w316, index=w315) -> (element=w314:string)
        n208 = Format Into String(format string="%s   %dfps   %d%%", w314, w313, w312) -> (resulting string=w319:string)  [unwired: 2 in, 1 out]
        n209 = Build Array(w319) -> (w320:string[])
        n210 = property on="DB Camera Config" class="Bool (strict)"("Strings [4]"=w320) -> ()  [unwired: 2 in, 2 out]
      }
      event "Motor.Enable": Value Change {
        # "When the test mode otor enable helper is set, update that\ntree row item's value"
        n211 = event-data() -> ("NewVal"=w328:bool)  [unwired: 1 in]
        n212 = Unbundle("Motor") -> ("Value"=w327:dbl)  [unwired: 1 out]
        n213 = Select(t=w327, s=w328, f=0.0) -> (s? t:f=w325:dbl)
        n214 = call <vilib>:"NT Write Number.vi"("Numeric"=w325, "Name"=w324) -> ()  [unwired: 9 in, 1 out]
      }
      event "Test Slider": Value Change {
        # "When the test mode slider helper is set, update that\ntree row item's value"
        n215 = event-data() -> ("NewVal"=w331:dbl)  [unwired: 1 in]
        n216 = call <vilib>:"NT Write Number.vi"("Numeric"=w331, "Name"=w332) -> ()  [unwired: 9 in, 1 out]
      }
      event "On/Off": Value Change {
        # "When the test mode on/off helper value is set, update that\ntree row item's value"
        n217 = event-data() -> ("NewVal"=w336:bool)  [unwired: 1 in]
        n218 = Boolean To (0,1)(Boolean=w336) -> (0, 1=w335:i16)
        n219 = call <vilib>:"NT Write Number.vi"("Numeric"=w335, "Name"=w334) -> ()  [unwired: 9 in, 1 out]
      }
      event "Rev/Fwd": Value Change {
        # "When the test mode helper value for relays is set, update that\ntree row item's value"
        n220 = event-data() -> ("NewVal.Forward"=w344:bool, "NewVal.Reverse"=w343:bool)  [unwired: 1 in]
        n221 = Boolean To (0,1)(Boolean=w344) -> (0, 1=w340:i16)
        n222 = Boolean To (0,1)(Boolean=w343) -> (0, 1=w342:i16)
        n223 = Negate(x=w342) -> (-x=w341:i16)
        n224 = Add(x=w340, y=w341) -> (x+y=w339:i16)
        n225 = call <vilib>:"NT Write Number.vi"("Numeric"=w339, "Name"=w338) -> ()  [unwired: 9 in, 1 out]
      }
      event "Test Ring": Value Change {
        # "When a test mode helper value is selected from the ring,\nset the tree item's variable to the string value"
        n226 = event-data() -> ("NewVal"=w348:u16)  [unwired: 1 in]
        n227 = property on="Test Ring" class="Ring (strict)"() -> ("Strings []"=w349:string[])  [unwired: 2 in, 2 out]
        n228 = Index Array(array=w349, index=w348) -> (element=w347:string)
        n229 = call <vilib>:"NT Write String.vi"("String"=w347, "Name"=w346) -> ()  [unwired: 9 in, 1 out]
      }
      event "Rec Mode": Value Change {
        # "Update globals for recording mode and path to read log from.\nClear when logging and let NetworkTables set path for vision to\nuse."
        n230 = event-data() -> ("NewVal"=w357:enum32{"Stop", "Record", "Playback"})  [unwired: 1 in]
        n231 = global write "WPI_DashboardLogging Global.vi" "Logging Filename"(path "") -> ()
        n232 = case shown="\"Playback\"" w357 {
          tunnel: w356 -> [_ w359 w367]
          tunnel: [_ _ w366] -> w353
          tunnel: [_ _ w365] -> _
          tunnel: w351 -> [_ _ w363]
          tunnel: cluster{i32, i32} {-250, 170} -> [_ _ w362]
          tunnel: [_ _ T28 {"Image Size"=TRUE, "Image Type"=TRUE, "Pixel Value"=TRUE, "ROI Information"=TRUE, "Zoom Factor"=FALSE} ("Image Information Shown:All Elements")] -> _
          tunnel: [_ _ TRUE ("Zoom Factor")] -> _
          frame Default {
          }
          frame "Stop", "Record" {
            # "Place Window too"
            n233 = invoke class="VI" method="FP.Close"(reference=w359) -> (reference out=w358:refnum<vi>)  [unwired: 2 in, 2 out]
            n234 = invoke class="VI" method="Abort VI"(reference=w358) -> ()  [unwired: 2 in, 3 out]
          }
          frame "Playback" {
            n235 = call "Open Playback Panel.vi"("Offset"=w362, "DB VI Ref"=w363, "Playback in"=w367) -> ("Playback out"=w364:refnum<vi>)  [unwired: 8 in]
            n236 = register-events(w364) -> (reference out=w366:refnum<event-registration>, error out=w365:errorcluster)  [unwired: 2 in]
          }
        }
        n237 = global write "WPI_DashboardLogging Global.vi" "Recording"(w357) -> ()
        n238 = call <vilib>:"WPI_DashboardNT Log FieldName Cache.vi"("Operation"=enum16{"Lookup/Add", "Index", "Clear"}."Clear") -> ()  [unwired: 8 in, 3 out]
      }
      event Panel Close {
        w368 = enum32{"Stop", "Record", "Playback"}."Stop" ("Rec Mode")
        # "Playback window has been closed, abort"
        n239 = event-data() -> ()  [unwired: 1 in, 4 out]
        n240 = local write "Rec Mode"(w368) -> ()
        n241 = global write "WPI_DashboardLogging Global.vi" "Recording"(w368) -> ()
      }
      event Panel Close {
        # "Abort playback window and ourself"
        n242 = event-data() -> ()  [unwired: 1 in, 4 out]
        n243 = invoke class="VI" method="FP.Close"(reference=w373) -> (reference out=w372:refnum<vi>)  [unwired: 2 in, 2 out]
        n244 = invoke class="VI" method="Abort VI"(reference=w372) -> (error out=w371:errorcluster)  [unwired: 2 in, 2 out]
        n245 = invoke class="VI" method="Abort VI"(error in=w371) -> ()  [unwired: 2 in, 3 out]
      }
      event "Vision": Value Change {
        # "Enable/Disable Compression slider.\nHW USB is hard-coded into the camera"
        n246 = event-data() -> ("NewVal"=w379:u16)  [unwired: 1 in]
        n247 = Equal?(x=w379, y=u32 2 ("milliseconds to wait")) -> (x = y?=w377:bool)
        n248 = Select(t=T29."Disabled and Grayed Out" ("Disabled"), s=w377, f=T29."Enabled" ("Disabled")) -> (s? t:f=w374:T29)
        n249 = property on="Compression" class="Slide (strict)"("DisabledEnum"=w374) -> ()  [unwired: 2 in, 2 out]
      }
    }
  }
  n250 = while {
    tunnel: w43 -> [w382]
    i -> [w385]
    stop <- FALSE stop-if-true
    n251 = Wait (ms)(milliseconds to wait=u32 100) -> ()  [unwired: 1 out]
    n252 = case shown="\"Playback\"" "Rec Mode" {
      tunnel: w385 -> [_ _ w400]
      tunnel: [u32 2829099 ("Base Color") u32 11141120 ("Target Color") w389] -> w381
      frame "Stop", Default {
        # "Reset the color, extra updates don't cost much"
      }
      frame "Record" {
      }
      frame "Playback" {
        # "Playback"
        n253 = Quotient & Remainder(x=w400, y=u32 50 ("milliseconds to wait")) -> (x-y*floor(x/y)=w396:u32)  [unwired: 1 out]
        n254 = Divide(x=w396, y=u32 50 ("milliseconds to wait")) -> (x/y=w393:dbl)
        n255 = Multiply(x=6.283185307179586, y=w393) -> (x*y=w398:dbl)
        n256 = Sine(x=w398) -> (sin(x)=w397:dbl)
        n257 = Absolute Value(x=w397) -> (abs(x)=w390:dbl)
        n258 = call "Interpolate RGB Color.vi"("Proportion"=w390, "Target Color"=u32 30976, "Base Color"=u32 2829099) -> ("Result Color"=w389:u32)  [unwired: 8 in]
      }
    }
    n259 = property class="Pane"(reference=w382, "PaneColor"=w381) -> ()  [unwired: 1 in, 2 out]
  }
  n260 = call "IMAQ Create"("Image Name"="Masked Image", "Image Type"=w6) -> ("New Image"=w4:T1)  [unwired: 2 in, 2 out]
  n261 = call "IMAQ Create"("Image Name"="Dashboard Image", "Image Type"=w56) -> ("New Image"=w7:T1, "error out"=w54:errorcluster)  [unwired: 2 in, 1 out]
  n262 = while {
    tunnel: w7 -> [w411]
    tunnel: w54 -> [_]
    tunnel: [w412] -> _
    tunnel: w4 -> [w402]
    tunnel: w3 -> [w401]
    i -> [w412]
    stop <- FALSE stop-if-true
    n263 = local read "Rec Mode"() -> (w406:enum32{"Stop", "Record", "Playback"})
    n264 = call <vilib>:"WPI_CameraRead MJPG for Dashboard.vi"("Camera Settings"="Camera Settings", "Rec Mode"=w406, "Camera IP"="10.22.83.11", "Camera Mode"="Vision", "Refnum in"=w411) -> ("Active"=w410:bool, "Refnum out"=w403:T1, "FPS"=w409:dbl, "Bandwidth (Mbps)"=w408:dbl)  [unwired: 3 in]
    n265 = case shown="True" w410 {
      tunnel: w403 -> [_ w426]
      tunnel: w408 -> [_ w454]
      tunnel: w409 -> [_ w453]
      tunnel: w402 -> [_ w444]
      tunnel: w401 -> [_ w423]
      frame False {
        # "Sleep for 500ms"
        n266 = Wait Until Next ms Multiple(millisecond multiple=u32 500) -> ()  [unwired: 1 out]
      }
      frame True {
        w440 = 2.0  # Limit %
        w443 = 1.0  # Particles
        w425 = 4 ("Replace Value")
        w445 = u16 2 items=["RGB", "HSL", "HSV", "HSI"] ("Color Mode")
        # "Update Mbps LED"
        n267 = Unbundle("Tote Color") -> ("Hue"=w446:cluster{dbl, dbl}, "Sat"=w447:cluster{dbl, dbl}, "Val"=w448:cluster{dbl, dbl})
        n268 = case shown="4, 5" w454 {
          tunnel: [u32 6618880 ("Color Box") u32 16776722 ("Color Box") u32 16716800 ("Color Box")] -> w455
          frame Default {
          }
          frame 4, 5 {
          }
          frame 6.. {
          }
        }
        n269 = call "IMAQ Clear Overlay"("Image"=w426) -> ("error out"=w458:errorcluster)  [unwired: 2 in, 8 out]
        n270 = call "IMAQ ColorThreshold"("Blue or Luma or Val or Inten Range"=w448, "Replace Value"=w425, "Green or Sat Range"=w447, "Color Mode"=w445, "Red or Hue Range"=w446, "Image Dst"=w444, "Image Src"=w426) -> ("Image Dst Out"=w424:T1)  [unwired: 3 in, 1 out]
        "Image" <- w424
        n271 = Unbundle By Name(w458) -> ("status"=w459:bool)
        n272 = call "Sorted Particle Report 2015.vi"("Min Area Size %"=w440, "Particle Count Limit"=w443, "Pixel Measurements"=w423, "Image in"=w424) -> ("Sorted Data"=w441:dbl[][], "Particles"=→"Particles":i32)
        n273 = property on="Image Message" class="Str"("Visible"=w459) -> ()  [unwired: 2 in, 2 out]
        n274 = Bundle("Color Box"=w455, "Color Box"=w455) -> (w457:cluster{"Color Box":u32, "Color Box":u32})  [unwired: 1 out]
        n275 = Build Array(w457) -> (w456:cluster{"Color Box":u32, "Color Box":u32}[])
        n276 = call "Calculate Particle Scores.vi"("Pixel Value"=w425, "Limit Tests?"="Limit Tests?", "Aspect Fudge Factor"="Aspect Fudge Factor", "Sorted Data"=w441, "Image in"=w424) -> ("Scores"=w430:T31)  [unwired: 6 in]
        n277 = property on="Mbps 2" class="Bool (strict)"("Colors [4]"=w456) -> ()  [unwired: 2 in, 2 out]
        n278 = flat-sequence {
          tunnel: w430 -> [w460]
          tunnel: [w460] -> w429
          frame #0 {
            # "Evaluate and rank based\non goals and strategy?"
          }
        }
        n279 = Bundle("Red"="Red", "Blue"="Blue") -> (w433:T32)  [unwired: 1 in]
        n280 = call "Check for Carpet.vi"("Original Mask"=w424, "Original Color"=w426, "Carpet Colors"=w433, "Carpet Selector"="Carpet Color", "Combine Carpet Mask"="Show Carpet Mask", "Initial Scores"=w429) -> ("Updated Mask"=→"Masked":T1, "Updated Scores"=w422:T33)  [unwired: 4 in]
        n281 = Tick Count (ms)() -> (millisecond timer value=w451:u32)
        n282 = feedback #1() -> (w450:u32)  [unwired: 1 in]
        n283 = feedback-in #1(w451) -> ()
        n284 = Subtract(x=w451, y=w450) -> (x-y=→"ms to process":u32)
        n285 = call "Normalize Coordinates.vi"("Camera Type"="Camera Type", "Targets"=w422, "Image in"=w426) -> ("Found Totes"=w419:T9, "Sorted Scores"=→"Sorted Scores":T8)  [unwired: 7 in]
        "Detected Totes" <- w419
        n286 = call "Label Targets2.vi"("Score Threshold"="Score Threshold", "Annotate"="Annotate", "Targets"=w422, "Image in"=w426) -> ("Image out"=→"Original Image":T1)  [unwired: 7 in]
        n287 = Array To Cluster(array=w419) -> (cluster=w420:T34)
        n288 = Unbundle By Name(w420) -> ("Found Totes[0].Center"=w417:cluster{dbl, dbl})
        n289 = Unbundle(w417) -> (w416:dbl)  [unwired: 1 out]
        "Center" <- w416
        n290 = call-poly <vilib>:"SD Write Value.vi"("Numeric"=w416, "Name"="center") -> ()  [unwired: 8 in, 2 out]
        "Mbps" <- w454
        "fps" <- w453
      }
    }
  }
  n291 = TCP Create Listener(10:u16 1741 ("timeout ms (25000)")) -> (3:w8:refnum<k5>)  [unwired: 4 in, 2 out]
  n292 = while {
    tunnel: w8 -> [w465]
    stop <- FALSE stop-if-true
    n293 = TCP Wait On Listener(11:w465) -> (4:w464:refnum<k5>)  [unwired: 3 in, 4 out]
    n294 = local write "TCP"(w464) -> ()
  }
  n295 = property on="On/Off" class="Bool (strict)"("Visible"=w13) -> ()  [unwired: 2 in, 2 out]
  n296 = property on="Motor" class="Clust (strict)"("Visible"=w13) -> ()  [unwired: 2 in, 2 out]
  n297 = property on="Progress" class="Clust (strict)"("Visible"=w13) -> ()  [unwired: 2 in, 2 out]
  n298 = property on="Test Ring" class="Ring (strict)"("Visible"=w13) -> ()  [unwired: 2 in, 2 out]
  n299 = property on="Rev/Fwd" class="Clust (strict)"("Visible"=w13) -> ()  [unwired: 2 in, 2 out]
  n300 = property on="Camera Settings" class="Clust (strict)"("Visible"=w13) -> ()  [unwired: 2 in, 2 out]
  n301 = local write "DB Camera Config"(w13) -> ()
  n302 = global write "WPI_DashboardLogging Global.vi" "Recording"(w37) -> ()
  n303 = local write "Rec Mode"(w37) -> ()
